vi "AdvServoEventCreatePosChange.vi"(8 "error in (no error)":errorcluster, 11 "Device In":i32) -> (0 "error out":errorcluster, 2 "Event Registration Refnum Out":refnum<event-registration>, 3 "Device Out":i32)   [LabVIEW 2012]
uses:
  phidget21.dll
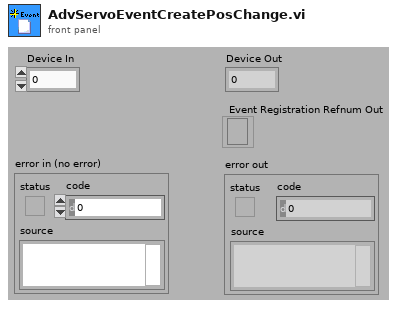
[diagram p1: front panel]
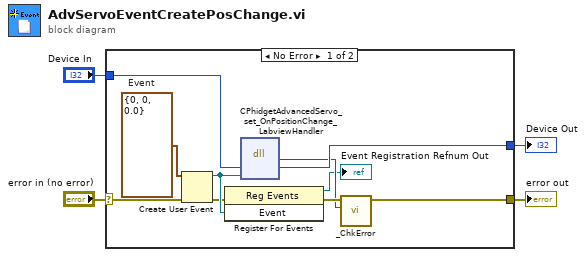
[diagram p0: block diagram]
diagram:
  n1 = case shown="No Error" "error in (no error)" {
    selector: "error in (no error)" -> [w13 w16]
    tunnel: [w7 w16] -> w3
    tunnel: "Device In" -> [w11 w15]
    tunnel: [w10 w15] -> w1
    frame No Error {
      w14 = cluster{"phid":i32, "index":i32, "Position":dbl} {"phid"=0, "index"=0, "Position"=0.0}  # Event
      n2 = Create User Event(user event datatype=w14, error in=w13) -> (user event=w12:refnum<user-event>, error out=w9:errorcluster)
      n3 = register-events(error in=w9, w12) -> (reference out=→"Event Registration Refnum Out":refnum<event-registration>, error out=w8:errorcluster)  [unwired: 1 in]
      n4 = dll-call lib="phidget21.*" fn="CPhidgetAdvancedServo_set_OnPositionChange_LabviewHandler"("phid"=w11, "Event"=w12) -> (w6:i32, "phid"=w10:i32)  [unwired: 4 in, 2 out]
      n5 = call "_ChkError.vi"("Return Code"=w6, "error in (no error)"=w8) -> ("error out"=w7:errorcluster)  [unwired: 9 in]
    }
    frame Error {
    }
  }
  "error out" <- w3
  "Device Out" <- w1
